vi "Max_get.vi"(9 "Current Max":dbl=16.775000000000002, 10 "on/off":bool=TRUE, 11 "Current Value":dbl=16.775000000000002) -> (2 "new max ping":bool, 3 "New Max":dbl=16.775000000000002)   [LabVIEW 2019]
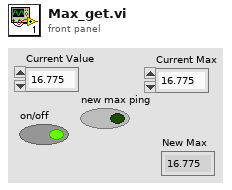
[diagram p1: front panel]
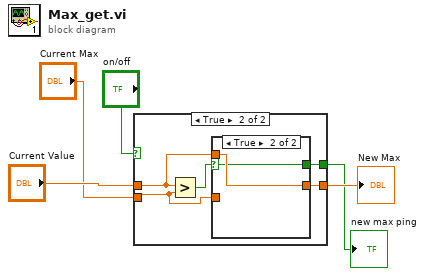
[diagram p0: block diagram]
diagram:
  n1 = case shown="True" "on/off" {
    selector: "on/off" -> [w6 _]
    tunnel: "Current Value" -> [w7 w11]
    tunnel: "Current Max" -> [_ w10]
    tunnel: [w7 w9] -> w2
    tunnel: [w6 w8] -> w1
    frame False {
    }
    frame True {
      n2 = Greater?(x=w11, y=w10) -> (0:w12:bool)
      n3 = case shown="True" w12 {
        selector: w12 -> [w13 w15]
        tunnel: w11 -> [_ w16]
        tunnel: w10 -> [w14 _]
        tunnel: [w14 w16] -> w9
        tunnel: [w13 w15] -> w8
        frame False {
        }
        frame True {
        }
      }
    }
  }
  "New Max" <- w2
  "new max ping" <- w1
